vi "Preference_global.vi"() -> ()   [LabVIEW 2011]
uses:
  Controls/Server_Comms.ctl
  Controls/EnFlo_Data_Folder_Setup.ctl
panel:
  in  "EnFlo_Data_Folder_Setup":T1="EnFlo_Data on Server"
  in  "User_Name":string
  in  "Default Source Establishment Time (s)":dbl=20.0
  out "Application:Version Number":string
  out "Operating System:Version Number":string
  out "Operating System:Name":string
  in  "% Error From First Calib":dbl=10.0 format="%.1f"
  in  "% Error From Previous Calib":dbl=0.5 format="%.1f"
  in  "Tunnel Speed Control":bool
  in  "SMTP server IP address":string="Run EnFlo Hub.vi"
  in  "Abs Press (mbar)":string="Run EnFlo Hub.vi"
  in  "Temperature":string="Run EnFlo Hub.vi"
  in  "Server port number":u32=3363
  in  "Server address":string="Please Run EnFlo Hub.vi"
  in  "LabVIEW Administrators":string[](array[string])
  in  "Unblock SMS":bool
  in  "Unblock Email":bool
  in  "Server Comms":T2
  in  "Rig Setup":string
  # "Deg C"
  # "Warning Levels for Autocalibration Changes"
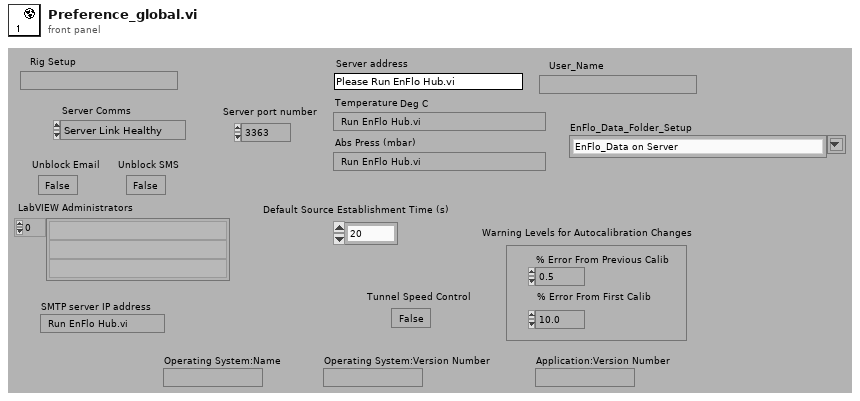
[diagram p1: front panel]
types:
  T1 = typedef "EnFlo_Data_Folder_Setup.ctl" = string
  T2 = typedef "Server_Comms.ctl" = enum16{"Server Link Healthy", "Do Not Link To Server"}
diagram:
